vi "Add Header To LogFile.vi"(8 "Error In":errorcluster, 10 "Header":string[](array[string]), 11 "LogClass In":refnum<class "LogsAbstract.lvclass">) -> (0 "Error Out":errorcluster, 3 "LogClass Out":refnum<class "LogsAbstract.lvclass">)   [LabVIEW 2019, in "LogsAbstract.lvlib" / "LogsAbstract.lvclass"]
uses:
  LogsAbstract.lvclass
  LogsAbstract.lvclass/LogsAbstract.ctl
  7e2e92b0-5b9d-495f-82df-d6128c21f1d1.vi
  7e2e92b0-5b9d-495f-82df-d6128c21f1d1.vi/314727cb-bc7d-47ca-a002-fa5ae311dc51.vi
  Accessors/Write LogPath.vi
  Accessors/Read LogPath.vi
  <vilib>/Utility/file.llb/Write Delimited Spreadsheet.vi
  <vilib>/Utility/file.llb/Write Delimited Spreadsheet (string).vi
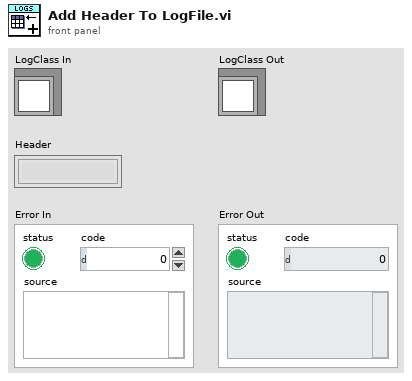
[diagram p1: front panel]
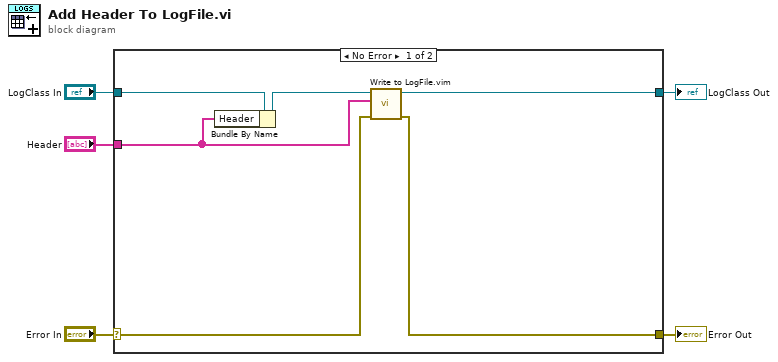
[diagram p0: block diagram]
diagram:
  n1 = case shown="No Error" "Error In" {
    selector: "Error In" -> [w9 w12]
    tunnel: [w8 w12] -> w4
    tunnel: "LogClass In" -> [w11 w13]
    tunnel: "Header" -> [w6 _]
    tunnel: [w10 w13] -> w1
    frame No Error {
      n2 = Bundle By Name(cluster=w11, "Header"=w6) -> (w7:refnum<class "LogsAbstract.lvclass">)
      n3 = call "Write to LogFile.vim"("Error In"=w9, "Data"=w6, "LogClass In"=w7) -> ("Error out"=w8:errorcluster, "LogClass Out"=w10:refnum<class "LogsAbstract.lvclass">)  [unwired: 7 in]
    }
    frame Error {
    }
  }
  "LogClass Out" <- w1
  "Error Out" <- w4
